vi "KeyenceCVX.Main.ChangeProgram.vi"(8 "error in":errorcluster, 10 "ChangeProgram.Data":T1, 11 "Data":T2) -> (0 "error out":errorcluster, 3 "Data out":T2)   [LabVIEW 2016]
uses:
  KeyenceCVX.Data.ctl
  KeyenceCVX.Data.Status.ctl
  KeyenceCVX.Data.Status.State.ctl
  KeyenceCVX.Data.Sets.ctl
  KeyenceCVX.CodeDetails.ctl
  KeyenceCVX.ChangeProgram.Data.ctl
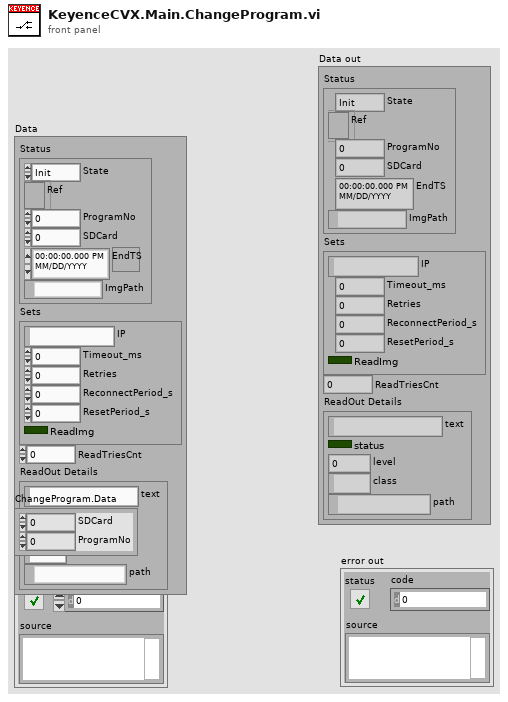
[diagram p1: front panel]
types:
  T1 = typedef "KeyenceCVX.ChangeProgram.Data.ctl" = cluster{"SDCard":u8, "ProgramNo":u16}
  T2 = typedef "KeyenceCVX.Data.ctl" = cluster{"Status":T3, "Sets":T5, "ReadTriesCnt":u8, "ReadOut Details":T6}
  T3 = typedef "KeyenceCVX.Data.Status.ctl" = cluster{"State":T4, "Ref":refnum<k5>, "ProgramNo":u16, "SDCard":u8, "EndTS":timestamp, "ImgPath":path}
  T4 = typedef "KeyenceCVX.Data.Status.State.ctl" = enum16{"Init", "Reset", "Idle", "Scan"}
  T5 = typedef "KeyenceCVX.Data.Sets.ctl" = cluster{"IP":string, "Timeout_ms":i32, "Retries":i32, "ReconnectPeriod_s":i32, "ResetPeriod_s":i32, "ReadImg":bool}
  T6 = typedef "KeyenceCVX.CodeDetails.ctl" = cluster{"text":string, "status":bool, "level":u8, "class":string, "path":path}
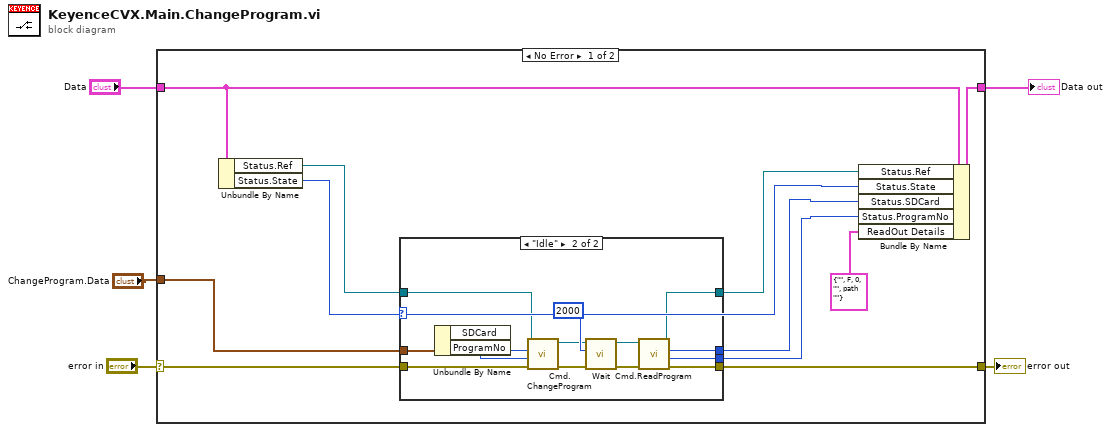
[diagram p0: block diagram]
diagram:
  n1 = case shown="No Error" "error in" {
    selector: "error in" -> [w16 w33]
    tunnel: [w12 w33] -> w4
    tunnel: "Data" -> [w14 w32]
    tunnel: [w11 w32] -> w2
    tunnel: "ChangeProgram.Data" -> [w10 _]
    frame No Error {
      n2 = Unbundle By Name(w14) -> ("Status.Ref"=w15:refnum<k5>, "Status.State"=w9:T4)
      n3 = case shown="\"Idle\"" w9 {
        tunnel: w15 -> [w18 w31]
        tunnel: w10 -> [_ w30]
        tunnel: w16 -> [w17 w29]
        tunnel: [w18 w26] -> w13
        tunnel: [w17 w23] -> w12
        tunnel: [_ w25] -> w8
        tunnel: [_ w24] -> w7
        frame Default {
        }
        frame "Idle" {
          n4 = Unbundle By Name(w30) -> ("SDCard"=w28:u8, "ProgramNo"=w27:u16)
          n5 = call "Cmd.ChangeProgram.vi"("error in"=w29, "Program"=w27, "SDCard"=w28, "cID in"=w31) -> ("error out"=w22:errorcluster, "cID out"=w19:refnum<k5>)  [unwired: 6 in]
          n6 = call "Wait.vi"("error in (no error)"=w22, "Time(ms)"=2000) -> ("error out"=w21:errorcluster)  [unwired: 9 in]
          n7 = call "Cmd.ReadProgram.vi"("error in"=w21, "cID in"=w19) -> ("error out"=w23:errorcluster, "ProgramNumber"=w24:u16, "SDCard"=w25:u8, "cID out"=w26:refnum<k5>)  [unwired: 6 in]
        }
      }
      n8 = Bundle By Name(cluster=w14, "Status.Ref"=w13, "Status.State"=w9, "Status.SDCard"=w8, "Status.ProgramNo"=w7, "ReadOut Details"=T6 {"text"="", "status"=FALSE, "level"=0, "class"="", "path"=path ""}) -> (w11:T2)
    }
    frame Error {
    }
  }
  "error out" <- w4
  "Data out" <- w2
